vi "SetSide.vi"(8 "error in (no error)":errorcluster, 9 "MazeSite":refnum<class "MazeSite.lvclass">, 10 "Direction":T1, 11 "Room in":refnum<class "Room.lvclass">) -> (0 "error out":errorcluster, 3 "Room out":refnum<class "Room.lvclass">)   [LabVIEW 2020, in "Room.lvclass"]
uses:
  Room.lvclass
  Direction.ctl
  MazeSite/MazeSite.lvclass
  Room.lvclass/Room.ctl
  Private/Property/side/Read side.vi
  Private/Property/side/Write side.vi
  Property/roomNumber/Read roomNumber.vi
  Support/Class/ConsoleOutput.lvclass
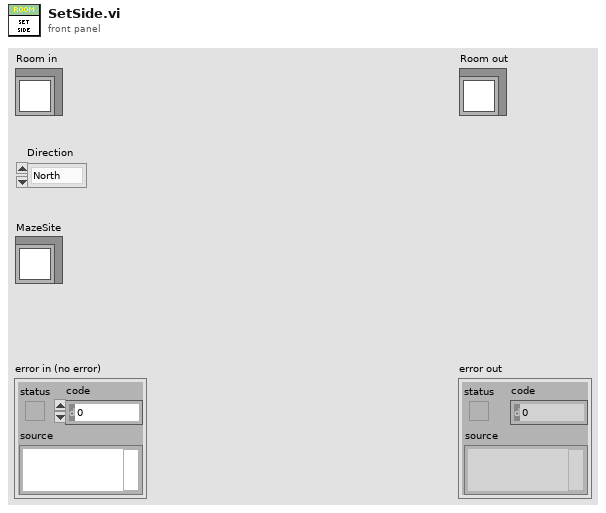
[diagram p1: front panel]
types:
  T1 = typedef "Direction.ctl" = enum32{"North", "South", "East", "West"}
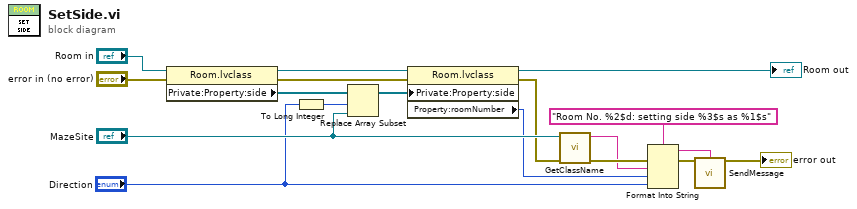
[diagram p0: block diagram]
diagram:
  n1 = property class="Room.lvclass"(reference="Room in", error in="error in (no error)") -> (reference out=w13:refnum<class "Room.lvclass">, error out=w12:errorcluster, "Private:Property:side"=w15:refnum<class "MazeSite.lvclass">[])
  n2 = To Long Integer(number="Direction") -> (32bit integer=w14:i32)
  n3 = Replace Array Subset(array=w15, new element="MazeSite", index=w14) -> (w11:refnum<class "MazeSite.lvclass">[])
  n4 = property class="Room.lvclass"(reference=w13, error in=w12, "Private:Property:side"=w11) -> (reference out=→"Room out":refnum<class "Room.lvclass">, error out=w7:errorcluster, "Property:roomNumber"=w2:i32)
  n5 = call "GetClassName.vi"("error in (no error)"=w7, "object"="MazeSite") -> ("error out"=w5:errorcluster, "Class Name"=w3:string)  [unwired: 8 in]
  n6 = Format Into String(format string="Room No. %2$d: setting side %3$s as %1$s" ("Message"), error in=w5, w3, w2, "Direction") -> (resulting string=w9:string, error out=w10:errorcluster)  [unwired: 1 in]
  n7 = call "SendMessage.vi"("Message"=w9, "error in (no error)"=w10) -> ("error out"=→"error out":errorcluster)  [unwired: 13 in]
